vi "RPT Comaristion.vi"(10 "True":bool) -> (1 "Fail":bool)   [LabVIEW 2015]
uses:
  Galobal variable_TI.vi
  Project Setup/Globle Variable/GR_Servo.vi
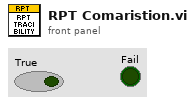
[diagram p1: front panel]
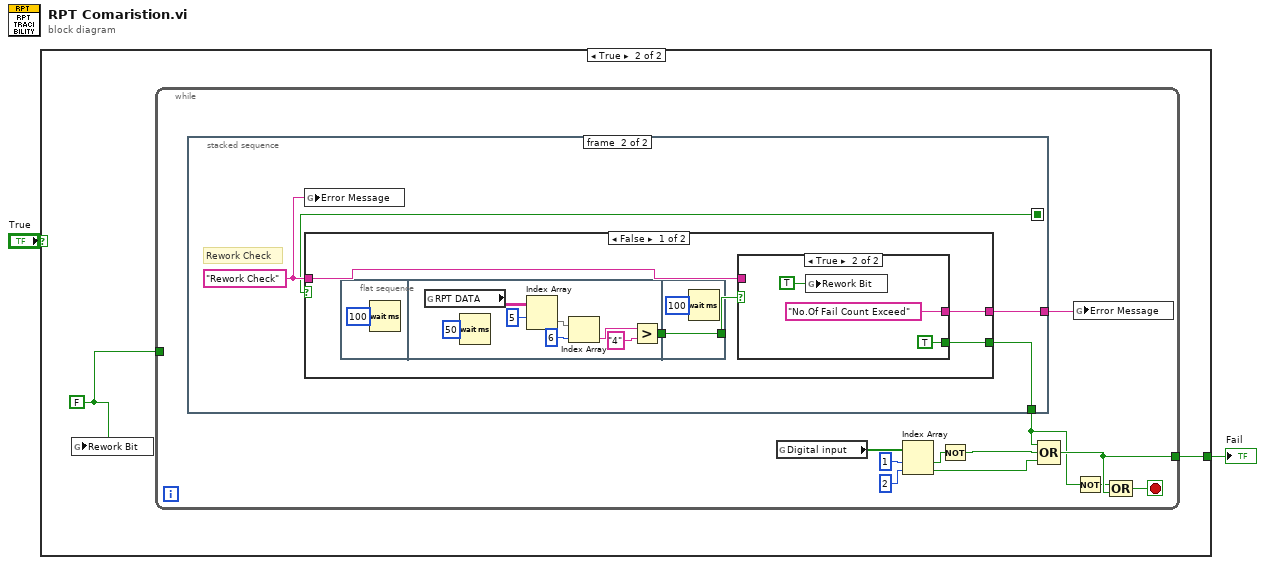
[diagram p0: block diagram]
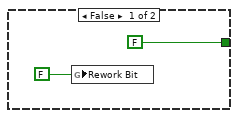
[diagram p2: hidden frame]
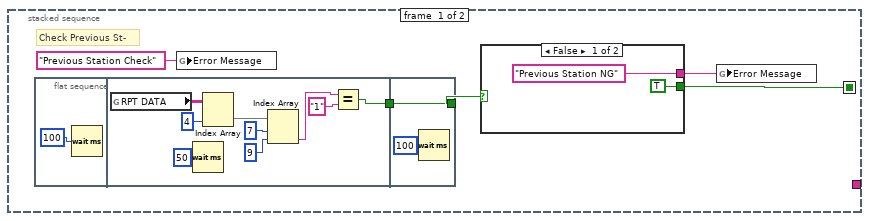
[diagram p3: hidden frame]
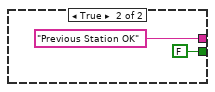
[diagram p4: hidden frame]
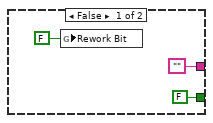
[diagram p5: hidden frame]
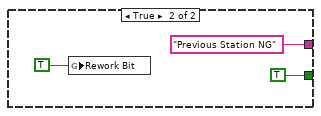
[diagram p6: hidden frame]
diagram:
  n1 = case shown="True" "True" {
    tunnel: [FALSE w6] -> w1
    frame False {
      n2 = global write "Galobal variable_TI.vi" "Rework Bit"(FALSE ("Rework bit")) -> ()
    }
    frame True {
      w5 = FALSE ("Rework bit")
      n3 = global write "Galobal variable_TI.vi" "Rework Bit"(w5) -> ()
      n4 = while {
        tunnel: [w10] -> w6
        tunnel: w5 -> [_]
        stop <- w11 stop-if-true
        n5 = stacked-sequence {
          seq-local: [w19 _] -> [_ w41]
          tunnel: [_ w40] -> w9
          tunnel: [_ w39] -> w8
          frame #0 {
            # "Check Previous St-"
            n6 = flat-sequence {
              tunnel: [w26] -> w18
              tunnel: [w34] -> w20
              tunnel: w18 -> [w34]
              frame #0 {
                n7 = Wait (ms)(milliseconds to wait=u32 100) -> ()  [unwired: 1 out]
              }
              frame #1 {
                n8 = global read "GR_Servo.vi" "RPT DATA"() -> (w27:string[][])
                n9 = Wait (ms)(milliseconds to wait=u32 50) -> ()  [unwired: 1 out]
                n10 = Index Array(array=w27, index (row)=4) -> (element=w29:string[])  [unwired: 1 in]
                n11 = Index Array(array=w29, index #1=7 ("index"), index #2=9 ("index")) -> (element #2=w32:string)  [unwired: 1 out]
                n12 = Equal?(x=w32, y="1") -> (x = y?=w26:bool)
              }
              frame #2 {
                n13 = Wait (ms)(milliseconds to wait=u32 100) -> ()  [unwired: 1 out]
              }
            }
            n14 = global write "GR_Servo.vi" "Error Message"("Previous Station Check") -> ()
            n15 = case shown="False" w20 {
              tunnel: ["Previous Station NG" "Previous Station OK"] -> w21
              tunnel: [TRUE FALSE] -> w19
              frame False {
              }
              frame True {
              }
            }
            n16 = global write "GR_Servo.vi" "Error Message"(w21) -> ()
          }
          frame #1 {
            w42 = "Rework Check"
            # "Rework Check"
            n17 = global write "GR_Servo.vi" "Error Message"(w42) -> ()
            n18 = case shown="False" w41 {
              tunnel: w42 -> [w46 _]
              tunnel: [w45 "Previous Station NG"] -> w40
              tunnel: [w44 TRUE] -> w39
              frame False {
                n19 = flat-sequence {
                  tunnel: [w51] -> w43
                  tunnel: [w58] -> w47
                  tunnel: w43 -> [w58]
                  frame #0 {
                    n20 = Wait (ms)(milliseconds to wait=u32 100) -> ()  [unwired: 1 out]
                  }
                  frame #1 {
                    n21 = global read "GR_Servo.vi" "RPT DATA"() -> (w53:string[][])
                    n22 = Wait (ms)(milliseconds to wait=u32 50) -> ()  [unwired: 1 out]
                    n23 = Index Array(array=w53, index (row)=5) -> (element=w56:string[])  [unwired: 1 in]
                    n24 = Index Array(array=w56, index=6) -> (element=w52:string)
                    n25 = Greater?(x=w52, y="4") -> (0:w51:bool)
                  }
                  frame #2 {
                    n26 = Wait (ms)(milliseconds to wait=u32 100) -> ()  [unwired: 1 out]
                  }
                }
                n27 = case shown="True" w47 {
                  tunnel: ["" "No.Of Fail Count Exceed"] -> w45
                  tunnel: w46 -> [_ _]
                  tunnel: [FALSE TRUE] -> w44
                  frame False {
                    n28 = global write "Galobal variable_TI.vi" "Rework Bit"(FALSE) -> ()
                  }
                  frame True {
                    n29 = global write "Galobal variable_TI.vi" "Rework Bit"(TRUE) -> ()
                  }
                }
              }
              frame True {
                n30 = global write "Galobal variable_TI.vi" "Rework Bit"(TRUE ("Rework bit")) -> ()
              }
            }
          }
        }
        n31 = global read "Galobal variable_TI.vi" "Digital input"() -> (w17:bool[])
        n32 = Index Array(array=w17, index #1=1 ("index"), index #2=2 ("index")) -> (element #1=w14:bool, element #2=w12:bool)
        n33 = Not(x=w14) -> (.not. x?=w13:bool)
        n34 = Compound Arithmetic op=OR(w8, w13, w12) -> (w10:bool)
        n35 = global write "GR_Servo.vi" "Error Message"(w9) -> ()
        n36 = Not(x=w8) -> (.not. x?=w7:bool)
        n37 = Compound Arithmetic op=OR(w7, w10) -> (w11:bool)
      }
    }
  }
  "Fail" <- w1
